vi "test pass.vi"(8 "error in (no error)":errorcluster, 11 "VI Tester Test in":refnum<class "VI Tester Test 6.lvclass">) -> (0 "error out":errorcluster, 3 "VI Tester Test out":refnum<class "VI Tester Test 6.lvclass">)   [LabVIEW 2020, in "VI Tester Test 6.lvclass"]
uses:
  VI Tester Test 6.lvclass
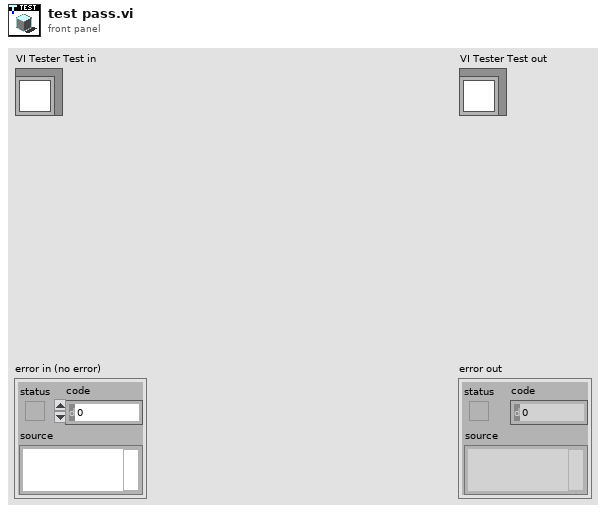
[diagram p1: front panel]
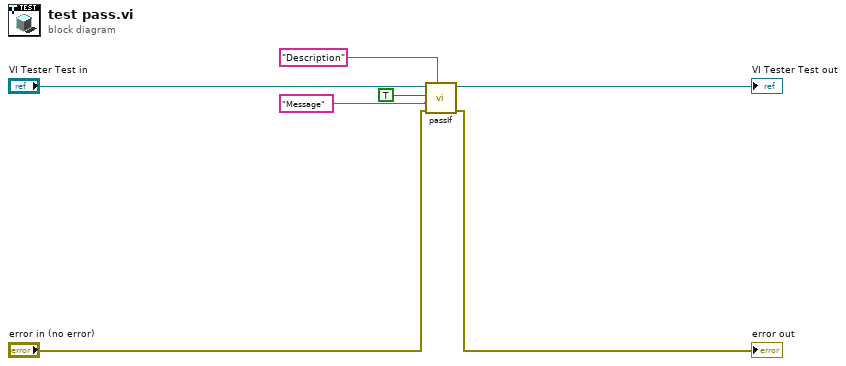
[diagram p0: block diagram]
diagram:
  n1 = call-dynamic "passIf.vi"("custom report message (\"\")"="Description" ("Description"), "error in (no error)"="error in (no error)", "message (\"\")"="Message" ("Message"), "pass"=TRUE ("Pass?"), "TestCase in"="VI Tester Test in") -> ("error out"=→"error out":errorcluster, "TestCase out"=→"VI Tester Test out":refnum<class "VI Tester Test 6.lvclass">)  [unwired: 5 in]
